vi "dfd_Get Integer Coefs.vi"(8 "error in (no error)":errorcluster, 11 "filter":T1={"mSRate_Fs"=1.0, "mSRate_Version"="1.0", "mSRate_Comments"="", "mSRate_OrgCoef"={"type"=enum."Undefined", "gain"=1.0, "coef a (k)"=[], "coef b (v)"=[]}, "mSRate_CurCoef"={"type"=enum."Undefined", "gain"=1.0, "coef a (k)"=[], "coef b (v)"=[]}, "mSRate_Quantized?"=FALSE, "mSRate_QCoef"={"type"=enum."Undefined", "gain"=1.0, "coef a (k)"=[], "coef b (v)"=[]}, "mSRate_QSettings"=[], "mSRate_Order"=0, "mSRate_Scaling"={"mSRate_ScaleByPowerOf2?"=FALSE, "mSRate_ScaleType"=enum."No Norm"}} {"mSRate_QSettings"."source" items=["Coef a/k"=0, "Coef b/v"=7, "Input"=1, "Output"=2, "Multiplicand"=3, "Product"=4, "Sum"=5, "Delay"=6, "Gain"=8]}) -> (0 "error out":errorcluster, 1 "int gain":cluster{"wl":i16, "integer":i32}, 2 "int coef a":cluster{"wl":i16, "integers":i32[]}, 3 "int coef b":cluster{"wl":i16, "integers":i32[]})   [LabVIEW 2017, in "NI_DigFilterLicensed.lvlib"]
uses:
  <vilib>/addons/Digital Filter Design/NI_DigFilterLicensed.lvlib
  <vilib>/addons/Digital Filter Design/_Objects.llb/DFD Filter Obj.ctl
  <vilib>/addons/Digital Filter Design/_Objects.llb/DFD Filter Coef.ctl
  <vilib>/addons/Digital Filter Design/_Objects.llb/DFD Filter Structure Type Selector.ctl
  <vilib>/addons/Digital Filter Design/_Objects.llb/dfd_Internal Quantization Settings.ctl
  <vilib>/addons/Digital Filter Design/_Objects.llb/dfd_Internal Quantization Srcs.ctl
  <vilib>/addons/Digital Filter Design/_Objects.llb/DFD Coef Norm Type.ctl
  <vilib>/addons/Digital Filter Design/NI_DigFilter_FXP.lvlib
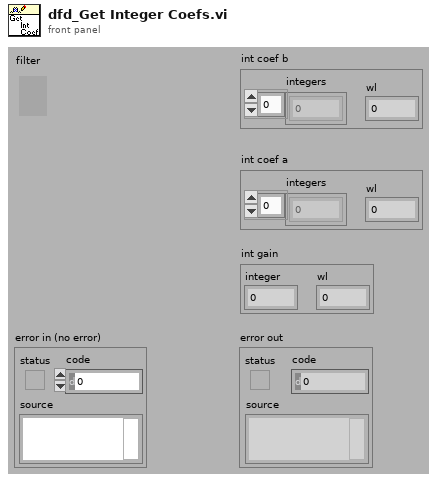
[diagram p1: front panel]
types:
  T1 = typedef "NI_DigFilterLicensed.lvlib/DFD Filter Obj.ctl" = cluster{"mSRate_Fs":dbl, "mSRate_Version":string, "mSRate_Comments":string, "mSRate_OrgCoef":T2, "mSRate_CurCoef":T2, "mSRate_Quantized?":bool, "mSRate_QCoef":T2, "mSRate_QSettings":T4[], "mSRate_Order":i32, "mSRate_Scaling":cluster{"mSRate_ScaleByPowerOf2?":bool, "mSRate_ScaleType":T6}}
  T2 = typedef "NI_DigFilterLicensed.lvlib/DFD Filter Coef.ctl" = cluster{"type":T3, "gain":dbl, "coef a (k)":dbl[], "coef b (v)":dbl[]}
  T3 = typedef "NI_DigFilterLicensed.lvlib/DFD Filter Structure Type Selector.ctl" = enum16{"Undefined", "FIR Direct Form", "FIR Direct Form Transposed", "FIR Symmetric", "FIR Antisymmetric", "IIR Direct Form I", "IIR Direct Form I Transposed", "IIR Direct Form II", "IIR Direct Form II Transposed", "IIR Cascaded Second Order Sections Form I", "IIR Cascaded Second Order Sections Form I Transposed", "IIR Cascaded Second Order Sections Form II", "IIR Cascaded Second Order Sections Form II Transposed", "Lattice Allpass (basic sections)", "Lattice Allpass (one multiplier sections)", "Lattice Allpass (normalized sections)", "Lattice AR (basic sections)", "Lattice AR (one multiplier sections)", "Lattice AR (normalized sections)", "Lattice MA (minimum phase)", "Lattice MA (maximum phase)", "Lattice ARMA (basic sections)", "Lattice ARMA (one multiplier sections)", "Lattice ARMA (normalized sections)"}
  T4 = typedef "NI_DigFilterLicensed.lvlib/dfd_Internal Quantization Settings.ctl" = cluster{"source":T5, "wl":i16, "iwl":i16, "overflow mode":enum16{"Saturation", "Wrap"}, "rounding mode":enum16{"Nearest", "Truncation"}, "signed?":bool}
  T5 = typedef "NI_DigFilterLicensed.lvlib/dfd_Internal Quantization Srcs.ctl" = u16
  T6 = typedef "NI_DigFilterLicensed.lvlib/DFD Coef Norm Type.ctl" = enum16{"No Norm", "Time Domain 1-Norm", "Time Domain 2-Norm", "Time Domain Inf-Norm"}
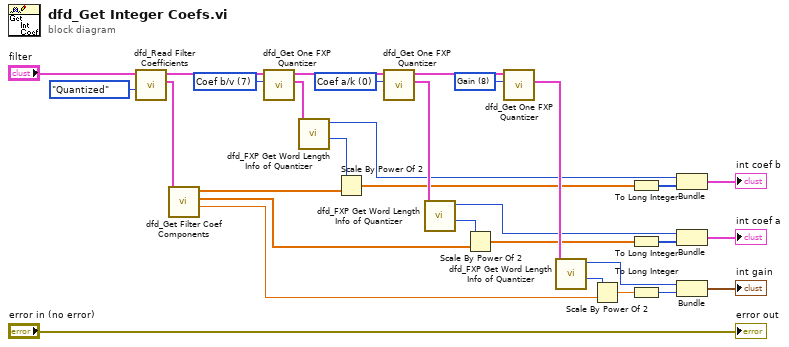
[diagram p0: block diagram]
diagram:
  w22 = T5 8 items=["Coef a/k"=0, "Coef b/v"=7, "Input"=1, "Output"=2, "Multiplicand"=3, "Product"=4, "Sum"=5, "Delay"=6, "Gain"=8] ("quantization source")
  w24 = T5 0 items=["Coef a/k"=0, "Coef b/v"=7, "Input"=1, "Output"=2, "Multiplicand"=3, "Product"=4, "Sum"=5, "Delay"=6, "Gain"=8] ("quantization source")
  w26 = T5 7 items=["Coef a/k"=0, "Coef b/v"=7, "Input"=1, "Output"=2, "Multiplicand"=3, "Product"=4, "Sum"=5, "Delay"=6, "Gain"=8] ("quantization source")
  n1 = call <vilib>:"dfd_Read Filter Coefficients.vi"("coef source"=enum16{"Original", "Current", "Quantized"}."Quantized", "filter in"="filter") -> ("filter coef"=w29:T2, "filter out"=w28:T1)  [unwired: 1 in, 7 out]
  n2 = call <vilib>:"dfd_Get Filter Coef Components.vi"("filter coef"=w29) -> ("gain"=w16:dbl, "coef a (k)"=w17:dbl[], "coef b (v)"=w18:dbl[])  [unwired: 1 in, 7 out]
  n3 = call <vilib>:"dfd_Get One FXP Quantizer.vi"("quantization source"=w26, "filter in"=w28) -> ("quantization settings"=w21:T4, "filter out"=w25:T1)  [unwired: 1 in, 7 out]
  n4 = call <vilib>:"dfd_FXP Get Word Length Info of Quantizer.vi"("quantization settings"=w21) -> ("fwl"=w15:i16, "wl"=w8:i16)  [unwired: 9 out]
  n5 = Scale By Power Of 2(n=w15, x=w18) -> (x*2^n=w12:dbl[])
  n6 = call <vilib>:"dfd_Get One FXP Quantizer.vi"("quantization source"=w24, "filter in"=w25) -> ("quantization settings"=w20:T4, "filter out"=w23:T1)  [unwired: 1 in, 7 out]
  n7 = call <vilib>:"dfd_FXP Get Word Length Info of Quantizer.vi"("quantization settings"=w20) -> ("fwl"=w14:i16, "wl"=w6:i16)  [unwired: 9 out]
  n8 = Scale By Power Of 2(n=w14, x=w17) -> (x*2^n=w11:dbl[])
  n9 = call <vilib>:"dfd_Get One FXP Quantizer.vi"("quantization source"=w22, "filter in"=w23) -> ("quantization settings"=w19:T4)  [unwired: 1 in, 8 out]
  n10 = call <vilib>:"dfd_FXP Get Word Length Info of Quantizer.vi"("quantization settings"=w19) -> ("fwl"=w13:i16, "wl"=w4:i16)  [unwired: 9 out]
  n11 = Scale By Power Of 2(n=w13, x=w16) -> (x*2^n=w10:dbl)
  n12 = To Long Integer(number=w12) -> (32bit integer=w9:i32[])
  n13 = To Long Integer(number=w11) -> (32bit integer=w7:i32[])
  n14 = To Long Integer(number=w10) -> (32bit integer=w5:i32)
  n15 = Bundle("wl"=w8, w9) -> (→"int coef b":cluster{"wl":i16, i32[]})  [unwired: 1 out]
  n16 = Bundle("wl"=w6, w7) -> (→"int coef a":cluster{"wl":i16, i32[]})  [unwired: 1 out]
  n17 = Bundle("wl"=w4, w5) -> (→"int gain":cluster{"wl":i16, i32})  [unwired: 1 out]
  "error out" <- "error in (no error)"
